vi "Write.vi"(8 "error in (no error)":errorcluster, 11 "Configuration in":refnum<class "Configuration.lvclass">) -> (0 "error out":errorcluster, 3 "Configuration out":refnum<class "Configuration.lvclass">)   [LabVIEW 2014, in "Configuration.lvlib" / "Configuration.lvclass"]
doc: "Write configuration data."
uses:
  Configuration.lvclass
  Configuration.lvclass/Configuration.ctl
  Interface/Interface.lvclass
  Section/Section.lvclass
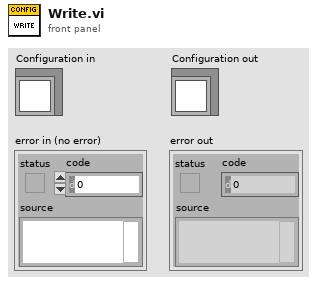
[diagram p1: front panel]
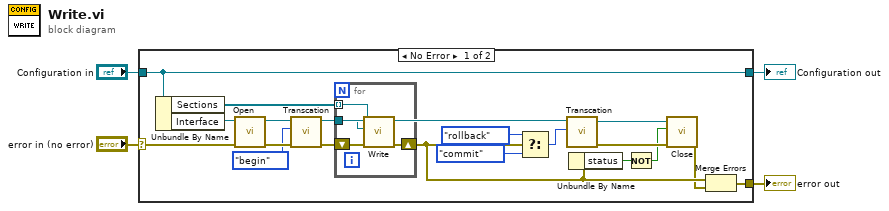
[diagram p0: block diagram]
diagram:
  n1 = case shown="No Error" "error in (no error)" {
    selector: "error in (no error)" -> [w22 w29]
    tunnel: [w9 w29] -> w3
    tunnel: [w21 w28] -> w1
    tunnel: "Configuration in" -> [w21 w28]
    frame No Error {
      n2 = Unbundle By Name(w21) -> ("Sections"=w20:refnum<class "Section.lvclass">[], "Interface"=w23:refnum<class "Interface.lvclass">)
      n3 = call-dynamic "Open.vi"("error in (no error)"=w22, "Interface in"=w23) -> ("error out"=w18:errorcluster, "Interface out"=w19:refnum<class "Interface.lvclass">)  [unwired: 8 in]
      n4 = call-dynamic "Transcation.vi"("error in (no error)"=w18, "Action"=enum16{"begin", "commit", "rollback"}."begin", "Interface in"=w19) -> ("error out"=w17:errorcluster, "Interface out"=w15:refnum<class "Interface.lvclass">)  [unwired: 7 in]
      n5 = for {
        tunnel: w20 -> [w27] mode=indexing
        shift-right: [w25] -> w8
        shift-left: w17 -> [w26]
        tunnel: w15 -> [w24]
        n6 = call "Write.vi"("error in (no error)"=w26, "Interface"=w24, "Section in"=w27) -> ("error out"=w25:errorcluster)  [unwired: 7 in, 1 out]
      }
      n7 = Select(t=enum16{"begin", "commit", "rollback"}."rollback" ("Action"), s=w8, f=enum16{"begin", "commit", "rollback"}."commit") -> (s? t:f=w11:enum16{"begin", "commit", "rollback"})
      n8 = call-dynamic "Transcation.vi"("Action"=w11, "Interface in"=w15) -> ("error out"=w10:errorcluster, "Interface out"=w14:refnum<class "Interface.lvclass">)  [unwired: 8 in]
      n9 = Unbundle By Name(w8) -> ("status"=w7:bool)
      n10 = Not(x=w7) -> (.not. x?=w6:bool)
      n11 = call-dynamic "Close.vi"("error in (no error)"=w10, "write if changed (T)"=w6, "Interface in"=w14) -> ("error out"=w5:errorcluster)  [unwired: 7 in, 1 out]
      n12 = Merge Errors(w8, w5) -> (w9:errorcluster)
    }
    frame Error {
    }
  }
  "error out" <- w3
  "Configuration out" <- w1
